vi "test Add Connections.vi"(8 "error in (no error)":errorcluster, 11 "TestCase in":refnum<class "Routing and Faulting Scripting Unit Tests.lvclass">) -> (0 "error out":errorcluster, 3 "TestCase out":refnum<class "Routing and Faulting Scripting Unit Tests.lvclass">)   [LabVIEW 2019, in "Routing and Faulting Scripting Unit Tests.lvclass"]
uses:
  Routing and Faulting Scripting Unit Tests.lvclass
  Shared/Routing State.ctl
  Shared/Connection.ctl
  Routing and Faulting Scripting Unit Tests.lvclass/Routing and Faulting Scripting Unit Tests.ctl
  <vilib>/addons/_JKI Toolkits/VI Tester/TestCase.llb/TestCase.lvclass
  Routing and Faulting Scripting.lvlib
  Shared/Routing and Faulting Shared.lvlib
  C:/Program Files (x86)/National Instruments/LabVIEW 2019/vi.lib/addons/_JKI Toolkits/VI Tester/TestCase.llb/TestCase.lvclass
panel:
  in  "Save?":bool
  out "Output Filename":string
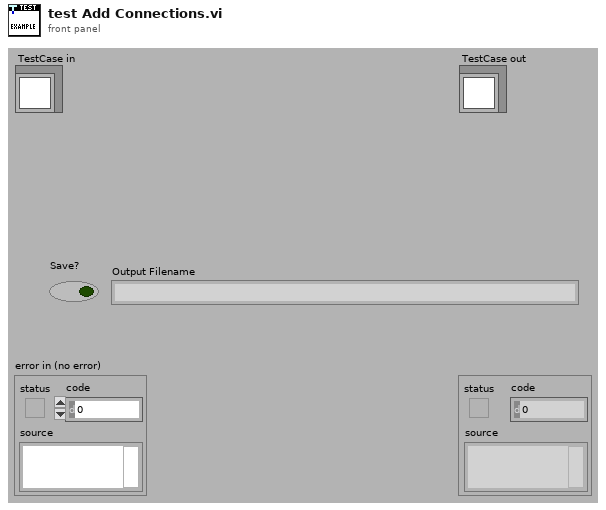
[diagram p1: front panel]
types:
  T1 = typedef "Routing and Faulting Shared.lvlib/Connection.ctl" = cluster{"Module":string, "Source":string, "Destination":string}
  T2 = typedef "Routing and Faulting Shared.lvlib/Routing State.ctl" = cluster{"Name":string, "Description":string, "Value":i32, "Connection List":T1[]}
  T3 = typedef "Custom Device API.lvlib/Custom Device Item Ref.ctl" = u64
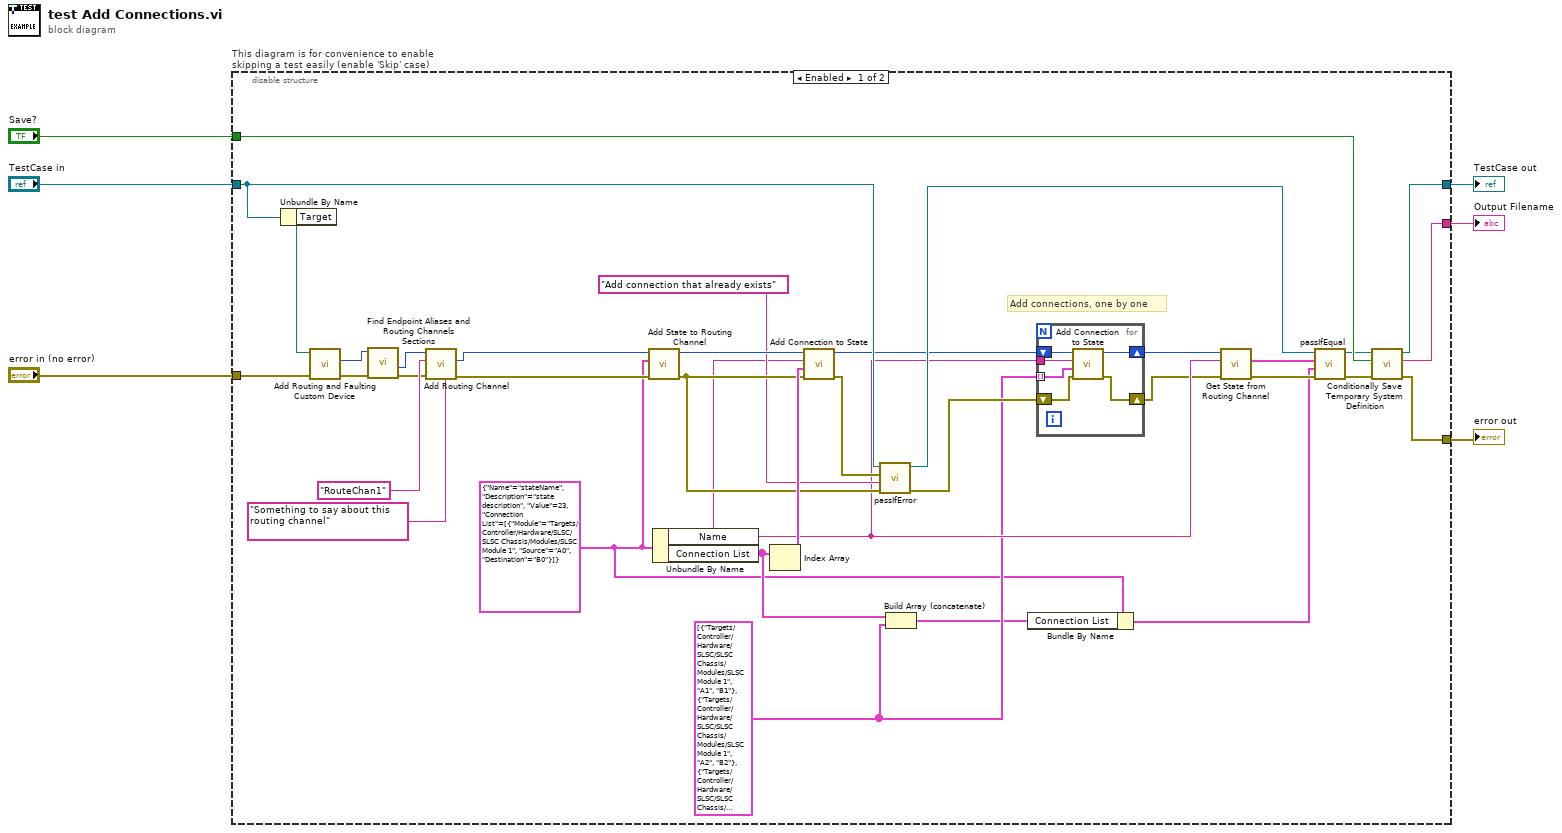
[diagram p0: block diagram]
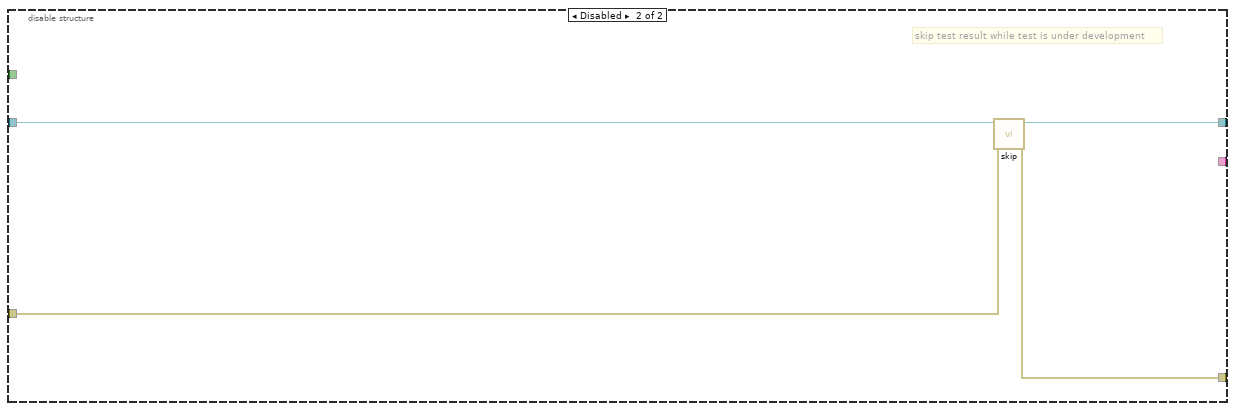
[diagram p2: hidden frame]
diagram:
  n1 = disable-structure "This diagram is for convenience to enable skipping a test easily (enable 'Skip' case)" shown="Enabled" {
    disable-tunnel: "TestCase in" -> [w26 w51]
    disable-tunnel: [w36 w49] -> w3
    disable-tunnel: [w40 w50] -> w5
    disable-tunnel: "error in (no error)" -> [w41 w48]
    disable-tunnel: [w39 _] -> w2
    disable-tunnel: "Save?" -> [w38 _]
    frame Enabled {
      w14 = T1[] [{"Module"="Targets/Controller/Hardware/SLSC/SLSC Chassis/Modules/SLSC Module 1", "Source"="A1", "Destination"="B1"}, {"Module"="Targets/Controller/Hardware/SLSC/SLSC Chassis/Modules/SLSC Module 1", "Source"="A2", "Destination"="B2"}, {"Module"="Targets/Controller/Hardware/SLSC/SLSC Chassis/Modules/SLSC Module 1", "Source"="A3", "Destination"="B3"}] ("connection list")
      w13 = T2 {"Name"="stateName", "Description"="state description", "Value"=23, "Connection List"=[{"Module"="Targets/Controller/Hardware/SLSC/SLSC Chassis/Modules/SLSC Module 1", "Source"="A0", "Destination"="B0"}]} ("Routing State")
      # "Add connections, one by one"
      n2 = Unbundle By Name(w26) -> ("Target"=w37:refnum<k24>)
      n3 = call "Add Routing and Faulting Custom Device.vi"("error in"=w41, "target in"=w37) -> ("error out"=w35:errorcluster, "routing and faulting custom device"=w9:T3)  [unwired: 7 in, 1 out]
      n4 = call "Find Endpoint Aliases and Routing Channels Sections.vi"("error in"=w35, "routing and faulting custom device in"=w9) -> ("error out"=w10:errorcluster, "routing channels"=w8:T3)  [unwired: 6 in, 2 out]
      n5 = call "Add Routing Channel.vi"("description"="Something to say about this routing channel" ("Description"), "error in"=w10, "channel name"="RouteChan1" ("Channel Name"), "routing channels in"=w8) -> ("error out"=w29:errorcluster, "routing channel"=w28:T3)  [unwired: 5 in, 1 out]
      n6 = call "Add State to Routing Channel.vi"("error in"=w29, "state and connections"=w13, "routing channel in"=w28) -> ("error out"=w22:errorcluster, "routing channel out"=w27:T3)  [unwired: 7 in]
      n7 = Unbundle By Name(w13) -> ("Name"=w20:string, "Connection List"=w15:T1[])
      n8 = Index Array(array=w15) -> (element=w24:T1)  [unwired: 1 in]
      n9 = call "Add Connection to State.vi"("error in"=w22, "connection"=w24, "state"=w20, "routing channel in"=w27) -> ("error out"=w23:errorcluster, "routing channel out"=w18:T3)  [unwired: 6 in]
      n10 = call-dynamic "passIfError.vi"("error in (no error)"=w22, "task (\"\")"="Add connection that already exists" ("task (\"\")"), "error"=w23, "TestCase in"=w26) -> ("error out"=w19:errorcluster, "TestCase out"=w25:refnum<class "Routing and Faulting Scripting Unit Tests.lvclass">)  [unwired: 6 in]
      n11 = Build Array (concatenate)(w15, w14) -> (w12:T1[])
      n12 = Bundle By Name(cluster=w13, "Connection List"=w12) -> (w11:T2)
      n13 = for {
        tunnel: w20 -> [w47]
        tunnel: w14 -> [w46] mode=indexing
        shift-right: [w42] -> w16
        shift-left: w19 -> [w45]
        shift-right: [w44] -> w17
        shift-left: w18 -> [w43]
        n14 = call "Add Connection to State.vi"("error in"=w45, "connection"=w46, "state"=w47, "routing channel in"=w43) -> ("error out"=w42:errorcluster, "routing channel out"=w44:T3)  [unwired: 6 in]
      }
      n15 = call "Get State from Routing Channel.vi"("error in"=w16, "state"=w20, "routing channel in"=w17) -> ("error out"=w32:errorcluster, "state and connections"=w31:T2)  [unwired: 6 in, 1 out]
      n16 = call-dynamic "passIfEqual.vi"("error in (no error)"=w32, "y"=w11, "x"=w31, "TestCase in"=w25) -> ("error out"=w34:errorcluster, "TestCase out"=w33:refnum<class "Routing and Faulting Scripting Unit Tests.lvclass">)  [unwired: 6 in]
      n17 = call "Conditionally Save Temporary System Definition.vi"("error in (no error)"=w34, "Save?"=w38, "Test Case"=w33) -> ("error out"=w40:errorcluster, "filename"=w39:string, "Test Case"=w36:refnum<class "Routing and Faulting Scripting Unit Tests.lvclass">)  [unwired: 6 in]
    }
    frame Disabled {
      # "skip test result while test is under development"
      n18 = call <vilib>:"skip.vi"("error in (no error)"=w48, "TestCase in"=w51) -> ("error out"=w50:errorcluster, "TestCase out"=w49:refnum<class "Routing and Faulting Scripting Unit Tests.lvclass">)  [unwired: 8 in]
    }
  }
  "error out" <- w5
  "TestCase out" <- w3
  "Output Filename" <- w2
